vi "Axis.vi"() -> ()   [LabVIEW 2019]
uses:
  <vilib>/picture/3D Picture Control/Object/Create Object (name).vi
  <vilib>/picture/3D Picture Control/NI_3D Picture Control.lvlib
panel:
  out "3D Picture":refnum<vi>(3d-picture)
  in  "Numeric":dbl
  in  "Boolean":bool
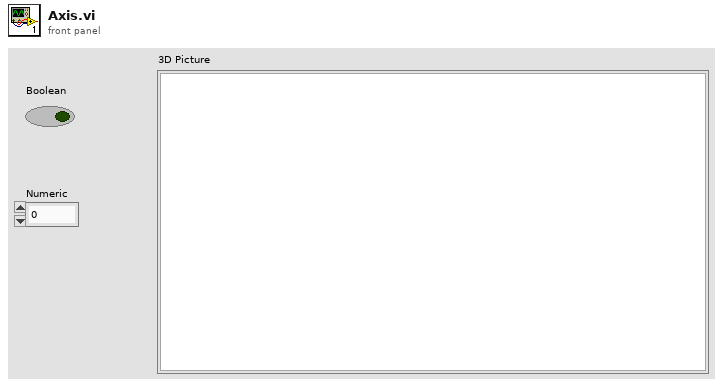
[diagram p1: front panel]
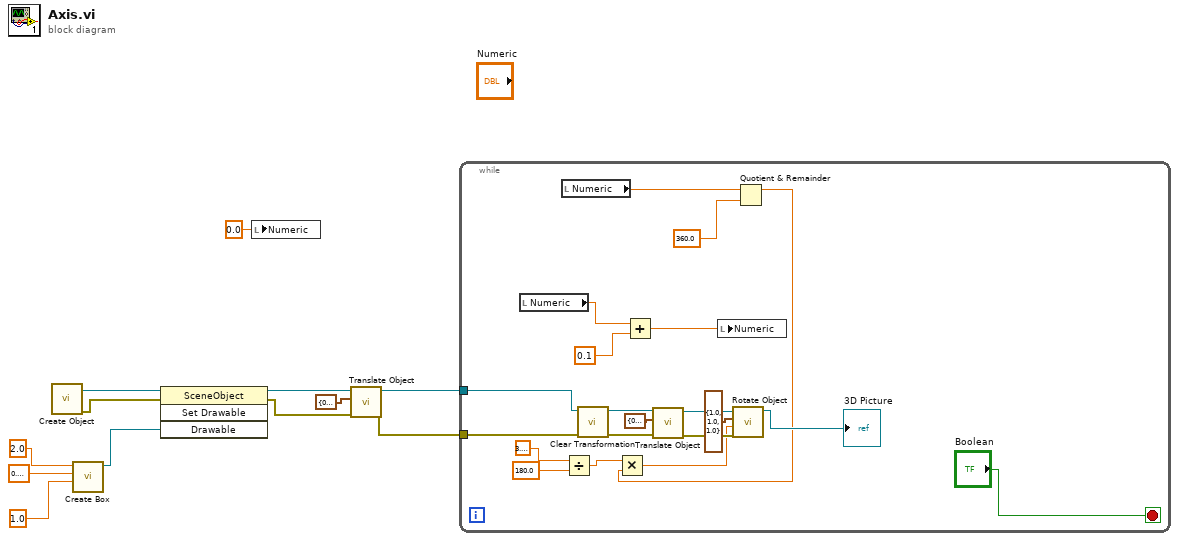
[diagram p0: block diagram]
diagram:
  n1 = call-poly <vilib>:"Create Object.vi"() -> ("error out"=w7:errorcluster, "Scene:New Object"=w8:refnum<vi>)  [unwired: 10 in]
  n2 = call <vilib>:"Create Box.vi"("Length Z"=sgl 1.0, "Length Y"=sgl 0.2, "Length X"=sgl 2.0) -> ("New Box Refnum"=w9:refnum<vi>)  [unwired: 7 in, 1 out]
  n3 = invoke class="SceneObject" method="Set Drawable"(reference=w8, error in=w7, "Drawable"=w9) -> (reference out=w6:refnum<vi>, error out=w5:errorcluster)  [unwired: 1 in, 2 out]
  n4 = local write "Numeric"(0.0 ("Numeric")) -> ()
  n5 = call <vilib>:"Translate Object.vi"("error in (no error)"=w5, "Translation"=cluster{"X":sgl, "Y":sgl, "Z":sgl} {"X"=0.0, "Y"=0.0, "Z"=0.0}, "Scene.Object In"=w6) -> ("error out"=w2:errorcluster, "Scene.Object Out"=w3:refnum<vi>)  [unwired: 7 in]
  n6 = while {
    tunnel: w3 -> [w19]
    tunnel: w2 -> [w18]
    stop <- "Boolean" stop-if-true
    n7 = local read "Numeric"() -> (w29:dbl)
    n8 = local read "Numeric"() -> (w30:dbl)
    n9 = Divide(x=3.141592653589793, y=180.0) -> (x/y=w15:dbl)
    n10 = call <vilib>:"Clear Transformation.vi"("error in (no error)"=w18, "Object Refnum In"=w19) -> ("error out"=w25:errorcluster, "Object Refnum Out"=w26:refnum<vi>)  [unwired: 8 in]
    n11 = Add(x=w29, y=0.1) -> (x+y=w27:dbl)
    n12 = call <vilib>:"Translate Object.vi"("error in (no error)"=w25, "Translation"=cluster{"X":sgl, "Y":sgl, "Z":sgl} {"X"=0.0, "Y"=0.0, "Z"=0.0}, "Scene.Object In"=w26) -> ("error out"=w22:errorcluster, "Scene.Object Out"=w23:refnum<vi>)  [unwired: 7 in]
    n13 = local write "Numeric"(w27) -> ()
    n14 = Quotient & Remainder(x=w30, y=360.0) -> (x-y*floor(x/y)=w13:dbl)  [unwired: 1 out]
    n15 = Multiply(x=w15, y=w13) -> (x*y=w14:dbl)
    n16 = call <vilib>:"Rotate Object.vi"("error in (no error)"=w22, "Angle"=w14, "Axis"=cluster{"X":sgl, "Y":sgl, "Z":sgl} {"X"=1.0, "Y"=1.0, "Z"=1.0}, "Scene.Object In"=w23) -> ("Scene.Object Out"=→"3D Picture":refnum<vi>)  [unwired: 6 in, 1 out]
  }
